vi "Helper Action.vi"(8 "error in (no error)":errorcluster, 9 "Message Data":variant, 10 "Message":string, 11 "Helper Loop In":refnum<class "Helper Loop.lvclass">) -> (0 "error out":errorcluster, 2 "Loop Period [ms]":u32=1000, 3 "Helper Loop Out":refnum<class "Helper Loop.lvclass">)   [LabVIEW 2020, in "Helper Loop.lvclass"]
doc: "The specific action implemented in the helper loop. Multiple different actions may be supported by using the Message and Message Data input to separate them. Any number of helper loops may run in parallell running the same or different actions. \nThe helper loop rate is controlled by the Loop Perid output of this method. \nIf this method throws an error, the helper loop will stop. The error will be sent to the error handler configured for the process. To stop it intentionally, the Stop Helper Loop.vi should be used. \nOne caveat with the helper loop is that it will have a copy of the object attributes as they were when the helper loop was started. If the attributes are updated, the helper loop will need to be restarted to refresh attributes."
uses:
  Helper Loop.lvclass
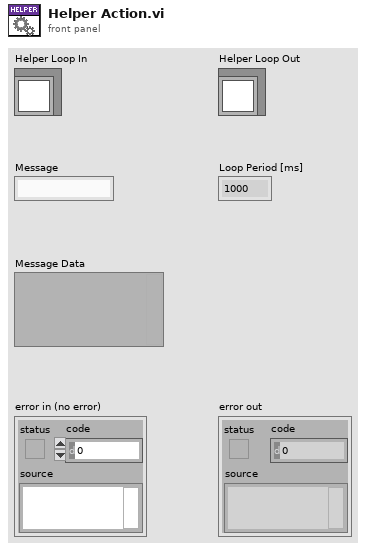
[diagram p1: front panel]
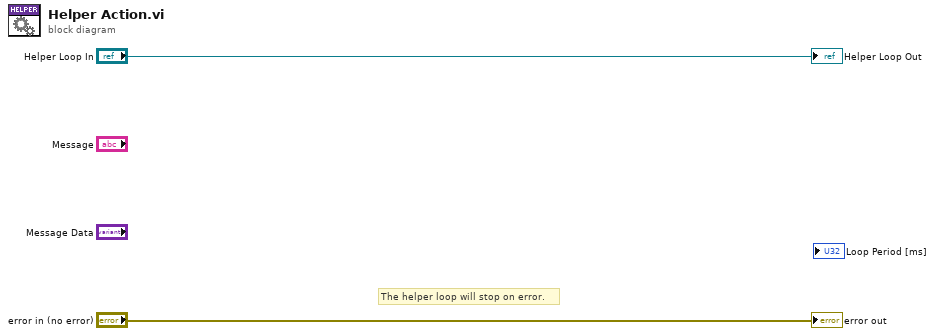
[diagram p0: block diagram]
diagram:
  # "The helper loop will stop on error."
  "error out" <- "error in (no error)"
  "Helper Loop Out" <- "Helper Loop In"
